vi "moveAxis.vi"(6 "Settings":T1, 7 "Channel":enum16{"X Axis", "Y Axis", "Z Axis"}(ring), 8 "error in":errorcluster, 9 "Acceleration":dbl=2.0, 10 "Velocity":dbl=2.0, 11 "Position (mm)":dbl=2.0) -> (0 "error out":errorcluster)   [LabVIEW 2017]
uses:
  Settings/Settings-Control.ctl
  <userlib>/ICNC/ICNC2.lvlib
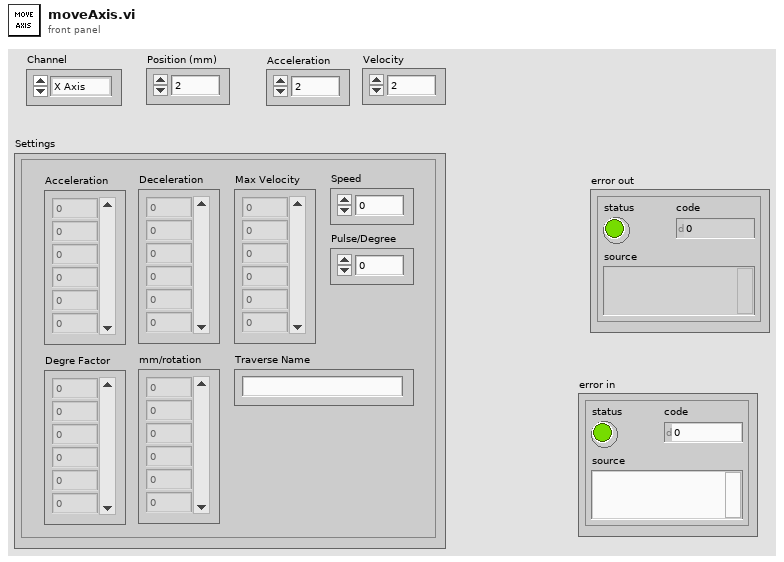
[diagram p1: front panel]
types:
  T1 = typedef "Settings-Control.ctl" = cluster{"Acceleration":dbl[], "Deceleration":dbl[], "Max Velocity":dbl[], "Speed":dbl, "Pulse/Degree":dbl, "Degre Factor":dbl[], "mm/rotation":dbl[], "Traverse Name":string}
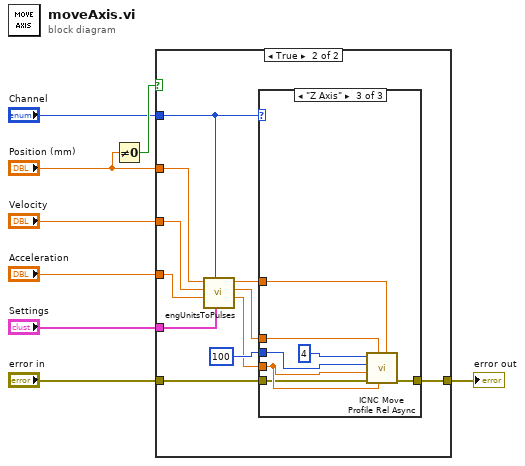
[diagram p0: block diagram]
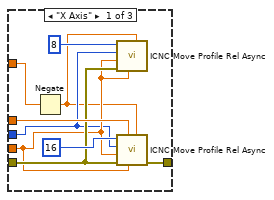
[diagram p3: hidden frame]
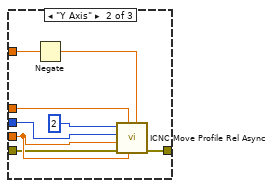
[diagram p4: hidden frame]
diagram:
  n1 = Not Equal To 0?(x="Position (mm)") -> (x != 0?=w8:bool)
  n2 = case shown="True" w8 {
    tunnel: "Position (mm)" -> [_ w15]
    tunnel: "Settings" -> [_ w14]
    tunnel: "Channel" -> [_ w16]
    tunnel: "Velocity" -> [_ w13]
    tunnel: "Acceleration" -> [_ w12]
    tunnel: "error in" -> [w9 w20]
    tunnel: [w9 w19] -> w1
    frame False {
    }
    frame True {
      n3 = call "engUnitsToPulses.vi"("Settings"=w14, "Channel"=w16, "Acceleration (mm/s^2)"=w12, "Velocity (mm/s)"=w13, "Position (mm)"=w15) -> ("kPulses /s^2"=w10:dbl, "Pulses /s"=w11:dbl, "Pulses"=w17:dbl)  [unwired: 4 in]
      n4 = case shown="\"Z Axis\"" w16 {
        tunnel: w10 -> [w24 w37 w44]
        tunnel: w11 -> [w29 w32 w39]
        tunnel: w20 -> [w25 w35 w42]
        tunnel: [w27 w36 w43] -> w19
        tunnel: 100 -> [w23 w34 w41]
        tunnel: w17 -> [w22 w31 w38]
        frame "X Axis" {
          n5 = Negate(x=w22) -> (-x=w21:dbl)
          n6 = call <userlib>:"ICNC Move Profile Rel Async.vi"("Distance"=w21, "Decel"=w24, "error in (no error)"=w25, "Accel"=w24, "FStartStop"=w23, "Axe"=u32 8) -> ()  [unwired: 4 in, 2 out]
          n7 = call <userlib>:"ICNC Move Profile Rel Async.vi"("Distance"=w21, "Decel"=w24, "Speed"=w29, "error in (no error)"=w25, "Accel"=w24, "FStartStop"=w23, "Axe"=u32 16) -> ("error out"=w27:errorcluster)  [unwired: 3 in, 1 out]
        }
        frame "Y Axis" {
          n8 = Negate(x=w31) -> (-x=w30:dbl)
          n9 = call <userlib>:"ICNC Move Profile Rel Async.vi"("Distance"=w30, "Decel"=w37, "Speed"=w32, "error in (no error)"=w35, "Accel"=w37, "FStartStop"=w34, "Axe"=u32 2) -> ("error out"=w36:errorcluster)  [unwired: 3 in, 1 out]
        }
        frame "Z Axis" {
          n10 = call <userlib>:"ICNC Move Profile Rel Async.vi"("Distance"=w38, "Decel"=w44, "Speed"=w39, "error in (no error)"=w42, "Accel"=w44, "FStartStop"=w41, "Axe"=u32 4) -> ("error out"=w43:errorcluster)  [unwired: 3 in, 1 out]
        }
      }
    }
  }
  "error out" <- w1
